vi "Simple P Controller.vi"(3 "Output Limit":dbl, 4 "Invert Output":bool, 5 "Proportional Gain (Kc)":dbl format="%_6g", 6 "Setpoint":dbl, 7 "Process Variable":dbl) -> (0 "Error Out":dbl, 1 "Output":dbl)   [LabVIEW 2012]
doc: "Determines the difference between the <b>setpoint</b> and <b>process variable</b> and determines the <b>output</b> by scaling that difference by the <b>proportional gain</b>. The output can be limited as well as inverted."
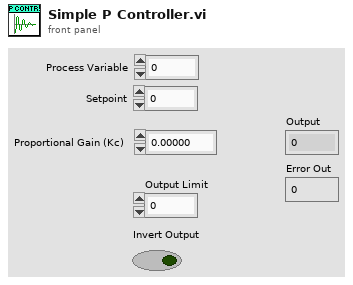
[diagram p1: front panel]
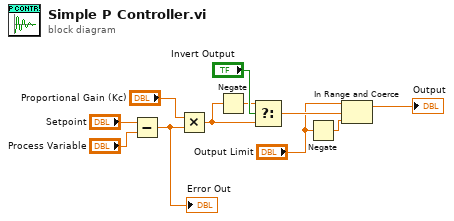
[diagram p0: block diagram]
diagram:
  n1 = Subtract(x="Setpoint", y="Process Variable") -> (x-y=w9:dbl)
  "Error Out" <- w9
  n2 = Multiply(x="Proportional Gain (Kc)", y=w9) -> (x*y=w5:dbl)
  n3 = Negate(x=w5) -> (-x=w6:dbl)
  n4 = Select(t=w6, s="Invert Output", f=w5) -> (s? t:f=w4:dbl)
  n5 = Negate(x="Output Limit") -> (-x=w1:dbl)
  n6 = In Range and Coerce(upper limit="Output Limit", x=w4, lower limit=w1) -> (coerced(x)=→"Output":dbl)  [unwired: 1 out]
